vi "Startup.vi"(8 "error in (no error)":errorcluster, 11 "Application in":refnum<class "Application.lvclass">) -> (0 "error out":errorcluster, 3 "Application out":refnum<class "Application.lvclass">)   [LabVIEW 2018, in "Application.lvlib" / "Application.lvclass"]
uses:
  Application.lvclass
  C:/Program Files/National Instruments/LabVIEW 2018/vi.lib/ActorFramework/Actor/Actor.lvclass
  User Interface/Splash Screen/Splash Screen.lvclass
  Application.lvclass/Application.ctl
  User Interface/Main Window/Main Window.lvclass
  Mode.ctl
  <vilib>/ActorFramework/Message Enqueuer/Message Enqueuer.lvclass/Message Enqueuer.ctl
  User Interface/Main Window Messages/Application Mode Change Msg/Application Mode Change Msg.lvclass/Application Mode Change Msg.ctl
  <vilib>/ActorFramework/Actor/Actor.lvclass/Actor.ctl
  User Interface/Splash Screen Messages/Update Status Msg/Update Status Msg.lvclass/Update Status Msg.ctl
  <vilib>/ActorFramework/Message Enqueuer/Enqueue.vi
  <vilib>/ActorFramework/Message Enqueuer/Init from Existing Queue.vi
  <vilib>/ActorFramework/Stop Msg/Stop Msg.lvclass
  C:/Program Files/National Instruments/LabVIEW 2018/vi.lib/ActorFramework/Message/Message.lvclass
  User Interface/Main Window Messages/Application Mode Change Msg/Application Mode Change Msg.lvclass
  User Interface/Splash Screen Messages/Update Status Msg/Update Status Msg.lvclass
  Resources/GLOBAL/GLOBAL Experiment Metadata.vi
  <vilib>/ActorFramework/Message Priority Queue/Priority Enqueue.vi
  <vilib>/ActorFramework/Message Enqueuer/Message Enqueuer.lvclass
  <vilib>/ActorFramework/Actor/Actor.lvclass
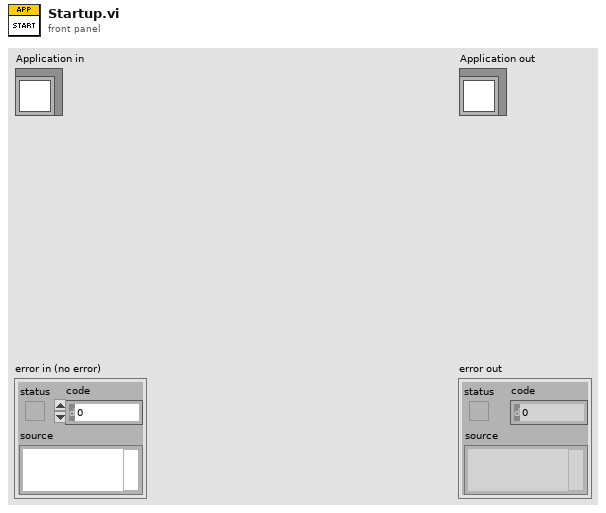
[diagram p1: front panel]
types:
  T1 = typedef "Mode.ctl" = enum16{"Idle", "Cancel", "Live", "Stream", "Autofocus", "Z-Stack"}
  T2 = typedef "Hardware Configuration.ctl" = cluster{"Shutters":T3[], "Stage Configuration":T4, "Microscope Configuration":T5, "Virtual Camera Configuration":T7, "Laser Configuration":T9[], "Fluidics Configuration":T10, "Installed Cameras":T11[], "Power Meter Configuration":cluster{"Power Meter Type":enum16{"Disabled", "Thorlabs", "Newport", "Coherent"}}}
  T3 = typedef "Shutter Configuration.ctl" = cluster{"IO Line":tag, "Name":string, "Wavelength":u16, "Max rate (Hz)":dbl}
  T4 = typedef "Stage Configuration.ctl" = cluster{"Serial Port":refnum<visa-resource-name>, "Forward Step (mm)":dbl, "Lane Length (mm)":dbl, "Lane Separation (mm)":dbl, "Stage Type":enum16{"Disabled", "ESP301", "Ti2", "Ludl", "ASI"}, "Autofocus Steps":i32, "Autofocus Range (um)":dbl, "Stage Limits":cluster{"Y Min":dbl, "Y Max":dbl, "X Min":dbl, "X Max":dbl}, "Slide (mm)":cluster{"top":dbl, "right":dbl, "width":dbl, "height":dbl}}
  T5 = typedef "Microscope Configuration.ctl" = cluster{"Serial Port":refnum<visa-resource-name>, "Microscope Type":T6, "Detection Settings":cluster{"Name":string, "Filter Position":u16, "Optical Path":u16}[]}
  T6 = typedef "Microscope Type.ctl" = enum16{"Disable", "TE2000", "Eclipse Ti", "Ti2"}
  T7 = typedef "Virtual Camera Configuration.ctl" = cluster{"Camera Type":T8, "Sync Line":tag}
  T8 = typedef "Camera Type.ctl" = enum16{"Hamamatsu"}
  T9 = typedef "Laser Configuration.ctl" = cluster{"Serial Port":refnum<visa-resource-name>, "Laser Type":enum16{"Disable", "Laser Quantum", "Coherent OBIS", "PRM1-Z8", "Coherent HOPS"}, "Polarizer Amplitude":dbl, "Polarizer Theta Zero":dbl, "Wavelength":u16}
  T10 = typedef "Pump Configuration.ctl" = cluster{"Fluidics present":bool}
  T11 = typedef "Physical Camera Assignment.ctl" = cluster{"Channel Name":string, "Camera Type":T8, "Serial Number":string, "Flip Vertically":bool, "Flip Horizontally":bool, "photonsPerCount":dbl, "wavelength":i16}
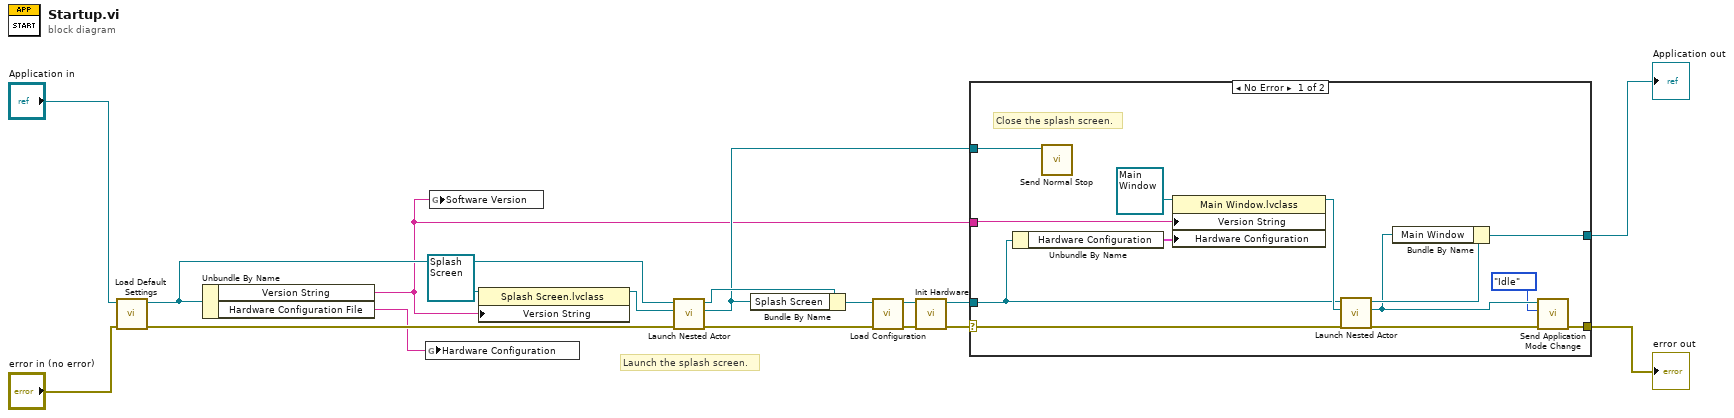
[diagram p0: block diagram]
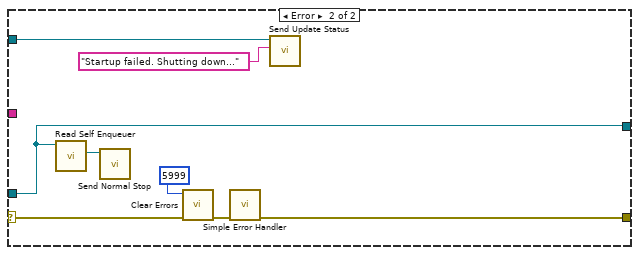
[diagram p2: hidden frame]
diagram:
  # "Launch the splash screen."
  n1 = call-dynamic "Load Default Settings.vi"("error in (no error)"="error in (no error)", "Application in"="Application in") -> ("error out"=w11:errorcluster, "Application out"=w15:refnum<class "Application.lvclass">)  [unwired: 8 in]
  n2 = Unbundle By Name(w15) -> ("Version String"=w7:string, "Hardware Configuration File"=w6:string)
  n3 = global write "GLOBAL Experiment Metadata.vi" "Hardware Configuration"(w6) -> ()
  n4 = global write "GLOBAL Experiment Metadata.vi" "Software Version"(w7) -> ()
  n5 = property class="Splash Screen.lvclass"(reference=refnum<class "Splash Screen.lvclass"> refnum ("Splash Screen.lvlib:Splash Screen.lvclass"), "Version String"=w7) -> (reference out=w16:refnum<class "Splash Screen.lvclass">)  [unwired: 1 in, 1 out]
  n6 = call <vilib>:"Launch Nested Actor.vi"("error in (no error)"=w11, "Nested Actor"=w16, "Caller Actor in"=w15) -> ("error out"=w5:errorcluster, "Nested Actor's Enqueuer"=w10:refnum<class "Message Enqueuer.lvclass">, "Caller Actor out"=w18:refnum<class "Application.lvclass">)  [unwired: 6 in]
  n7 = Bundle By Name(cluster=w18, "Splash Screen"=w10) -> (w13:refnum<class "Application.lvclass">)
  n8 = call-dynamic "Load Configuration.vi"("error in (no error)"=w5, "Application in"=w13) -> ("error out"=w9:errorcluster, "Application out"=w12:refnum<class "Application.lvclass">)  [unwired: 8 in]
  n9 = call-dynamic "Init Hardware.vi"("error in (no error)"=w9, "Application in"=w12) -> ("error out"=w8:errorcluster, "Application out"=w14:refnum<class "Application.lvclass">)  [unwired: 8 in]
  n10 = case shown="No Error" w8 {
    selector: w8 -> [w23 w33]
    tunnel: [w21 w36] -> w3
    tunnel: w7 -> [w30 _]
    tunnel: w14 -> [w28 w38]
    tunnel: [w27 w38] -> w4
    tunnel: w10 -> [w25 w39]
    frame No Error {
      # "Close the splash screen."
      n11 = Unbundle By Name(w28) -> ("Hardware Configuration"=w26:T2)
      n12 = call <vilib>:"Send Normal Stop.vi"("Message Enqueuer"=w25) -> ()  [unwired: 10 in, 1 out]
      n13 = property class="Main Window.lvclass"(reference=refnum<class "Main Window.lvclass"> refnum ("Main Window.lvlib:Main Window.lvclass"), "Version String"=w30, "Hardware Configuration"=w26) -> (reference out=w29:refnum<class "Main Window.lvclass">)  [unwired: 1 in, 1 out]
      n14 = call <vilib>:"Launch Nested Actor.vi"("error in (no error)"=w23, "Nested Actor"=w29, "Caller Actor in"=w28) -> ("error out"=w20:errorcluster, "Nested Actor's Enqueuer"=w22:refnum<class "Message Enqueuer.lvclass">, "Caller Actor out"=w24:refnum<class "Application.lvclass">)  [unwired: 6 in]
      n15 = Bundle By Name(cluster=w24, "Main Window"=w22) -> (w27:refnum<class "Application.lvclass">)
      n16 = call "Send Application Mode Change.vi"("error in (no error)"=w20, "Mode"=Mode."Idle", "Message Enqueuer"=w22) -> ("error out"=w21:errorcluster)  [unwired: 7 in, 1 out]
    }
    frame Error {
      n17 = call <vilib>:"Read Self Enqueuer.vi"("Actor"=w38) -> ("Self Enqueuer"=w37:refnum<class "Message Enqueuer.lvclass">)  [unwired: 10 in]
      n18 = call <vilib>:"Send Normal Stop.vi"("Message Enqueuer"=w37) -> ()  [unwired: 10 in, 1 out]
      n19 = call <vilib>:"Clear Errors.vi"("error in (no error)"=w33, "specific error code to clear (0: all)"=5999) -> ("error out"=w35:errorcluster)  [unwired: 4 in, 1 out]
      n20 = call <vilib>:"Simple Error Handler.vi"("error in (no error)"=w35) -> ("error out"=w36:errorcluster)  [unwired: 4 in, 4 out]
      n21 = call "Send Update Status.vi"("Status Message"="Startup failed. Shutting down...", "Message Enqueuer"=w39) -> ()  [unwired: 8 in, 2 out]
    }
  }
  "error out" <- w3
  "Application out" <- w4
